vi "Helmholtz2D_FEM_Assemble_Stiffness Mtrx.vi"(9 "area":dbl, 10 "Tri Y":dbl[](array[numeric]), 11 "Tri X":dbl[](array[numeric])) -> (3 "Stiffness Mtrx":dbl[][](array[numeric]))   [LabVIEW 2017, in "NI_PDE.lvlib"]
uses:
  <vilib>/gmath/NI_PDE.lvlib
  <vilib>/Analysis/baseanly.llb/Real Outer Product.vi
  <vilib>/Analysis/Matrix/Numeric/Add/Add - RM,RM.vi
  <vilib>/Analysis/NI_AALBase.lvlib
  <vilib>/Analysis/Matrix/NI_Matrix.lvlib
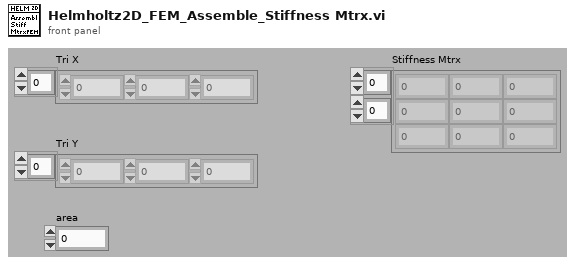
[diagram p1: front panel]
types:
  T1 = typedef "NI_Matrix.lvlib/RealMatrix.ctl" = dbl[][]
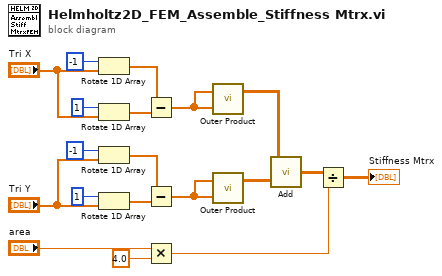
[diagram p0: block diagram]
diagram:
  n1 = Rotate 1D Array(1:"Tri X", 2:-1 ("n")) -> (0:w16:dbl[])
  n2 = Rotate 1D Array(1:"Tri X", 2:1 ("n")) -> (0:w15:dbl[])
  n3 = Rotate 1D Array(1:"Tri Y", 2:-1 ("n")) -> (0:w11:dbl[])
  n4 = Rotate 1D Array(1:"Tri Y", 2:1 ("n")) -> (0:w12:dbl[])
  n5 = Subtract(x=w16, y=w15) -> (x-y=w14:dbl[])
  n6 = Subtract(x=w11, y=w12) -> (x-y=w13:dbl[])
  n7 = Multiply(x="area", y=4.0) -> (x*y=w2:dbl)
  n8 = call-poly <vilib>:"Outer Product.vi"("Y Vector"=w14, "X Vector"=w14) -> ("Outer Product"=w7:T1)  [unwired: 1 out]
  n9 = call-poly <vilib>:"Outer Product.vi"("Y Vector"=w13, "X Vector"=w13) -> ("Outer Product"=w6:T1)  [unwired: 1 out]
  n10 = call-poly <vilib>:"Add.vi"("Real Matrix B"=w6, "Real Matrix A"=w7) -> ("A + B"=w3:T1)
  n11 = Divide(x=w3, y=w2) -> (x/y=→"Stiffness Mtrx":T1)
